vi "Open Base System Definition.vi"(8 "error in (no error)":errorcluster) -> (0 "error out":errorcluster, 3 "SystemDefinition":refnum<k24>)   [LabVIEW 2019, in "SLSC Switch Scripting System Tests.lvclass"]
uses:
  SLSC Switch Scripting System Tests.lvclass
  <vilib>/NI/VeriStand Custom Device Testing Tools/VeriStandTestUtilities/VeriStandTestUtilities.lvlib
  <userlib>/_OpenG.lib/file/file.llb/Append Path to Root if Relative - Scalar__ogtk.vi
  NationalInstruments.VeriStand.SystemDefinitionAPI
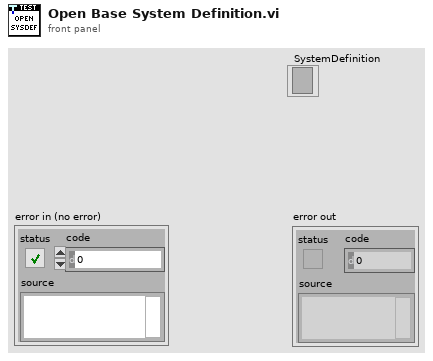
[diagram p1: front panel]
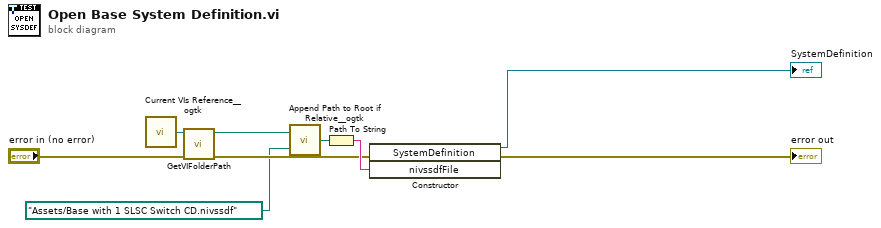
[diagram p0: block diagram]
diagram:
  n1 = call <userlib>:"Current VIs Reference__ogtk.vi"() -> ("Current VI's reference"=w3:refnum<vi>)  [unwired: 5 in]
  n2 = call <vilib>:"GetVIFolderPath.vi"("error in (no error)"="error in (no error)", "VI Reference in"=w3) -> ("error out"=w7:errorcluster, "VI Folder Path out"=w4:path)  [unwired: 8 in]
  n3 = call-poly <userlib>:"Append Path to Root if Relative__ogtk.vi"("Absolute or Relative Path"=path "Assets/Base with 1 SLSC Switch CD.nivssdf", "Root Path"=w4) -> ("Absolute or Appended Path"=w6:path)
  n4 = Path To String(path=w6) -> (string=w8:string)
  n5 = constructor class="SystemDefinition"(error in=w7, "nivssdfFile"=w8) -> (reference out=→"SystemDefinition":refnum<k24>, error out=→"error out":errorcluster)  [unwired: 2 in, 2 out]
